vi "NanotecSMCPDDriver.get library version.vi"() -> (0 "nameAndVersion":string)   [LabVIEW 2014, in "NanotecSMCPDDriver.lvlib"]
doc: "obtain name and version of a library as a string"
uses:
  NanotecSMCPDDriver.lvlib
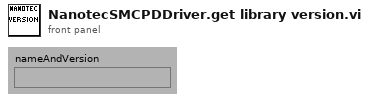
[diagram p1: front panel]
types:
  T1 = cluster{"Major":u16, "Minor":u16, "Fix":u16, "Build":u16}
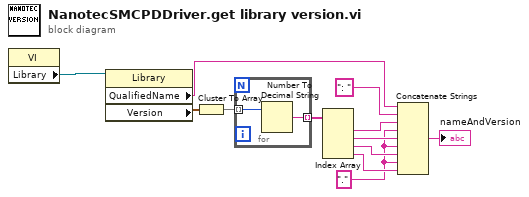
[diagram p0: block diagram]
diagram:
  w8 = "." ("string")
  n1 = property class="VI"() -> ("Library"=w1:refnum<vi>)  [unwired: 2 in, 2 out]
  n2 = property class="Library"(reference=w1) -> ("QualifiedName"=w5:string, "Version"=w2:T1)  [unwired: 1 in, 2 out]
  n3 = Cluster To Array(cluster=w2) -> (array=w3:u16[])
  n4 = for {
    tunnel: w3 -> [w14] mode=indexing
    tunnel: [w13] -> w4 mode=indexing
    n5 = Number To Decimal String(number=w14) -> (decimal integer string=w13:string)  [unwired: 1 in]
  }
  n6 = Index Array(array=w4) -> (element #1=w7:string, element #2=w9:string, element #3=w10:string, element #4=w11:string)  [unwired: 4 in]
  n7 = Concatenate Strings(w5, ": " ("string"), w7, w8, w9, w8, w10, w8, w11) -> (→"nameAndVersion":string)
